vi "Terminal-Global-StatusValues.vi"() -> ()   [LabVIEW 2014]
panel:
  out "主轴监测单元报警状态":bool
  out "陪试单元报警状态":bool
  out "试验单元报警状态":bool
  out "加载单元报警状态":bool
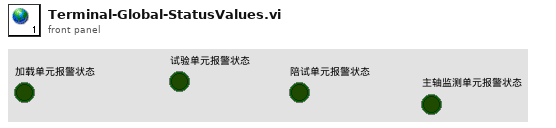
[diagram p1: front panel]
diagram:
